vi "S4GUI_002.vi"(7 "Tab ObsEng":enum32{"Obs", "CCD modes", "Eng"}(tab)) -> ()   [LabVIEW 2018] (continued)
                n2860 = call-dynamic "Read ref StatesQueue.vi"("error in (no error)"=w6117, "State Machine in"=w6116) -> ("error out"=w6127:errorcluster, "ref StatesQueue"=w6119:refnum<queue>, "State Machine out"=w6128:refnum<class "State Machine.lvclass">)  [unwired: 7 in]
                n2861 = Flush Queue(queue=w6119, error in (no error)=w6127) -> (queue out=w6118:refnum<queue>, error out=w6123:errorcluster)  [unwired: 1 out]
                n2862 = Enqueue Element(queue=w6118, element=u32 300 ("State"), error in (no error)=w6123) -> (queue out=w6126:refnum<queue>, error out=w6122:errorcluster)  [unwired: 1 in, 1 out]
                n2863 = Enqueue Element(queue=w6126, element=u32 60 ("State"), error in (no error)=w6122) -> (queue out=w6125:refnum<queue>, error out=w6124:errorcluster)  [unwired: 1 in, 1 out]
                n2864 = call-dynamic "Write ref StatesQueue.vi"("error in (no error)"=w6124, "ref StatesQueue"=w6125, "State Machine in"=w6128) -> ("error out"=w6114:errorcluster, "State Machine out"=w6115:refnum<class "State Machine.lvclass">)  [unwired: 7 in]
                n2865 = call-dynamic "Write State.vi"("error in (no error)"=w6114, "State"=0, "State Machine in"=w6115) -> ("error out"=w6131:errorcluster, "State Machine out"=w6134:refnum<class "State Machine.lvclass">)  [unwired: 7 in]
                n2866 = call-dynamic "Write State Machine.vi"("error in (no error)"=w6131, "State Machine.lvclass"=w6134, "Device in"=w6133) -> ("error out"=w6136:errorcluster, "Device out"=w6135:refnum<class "Channel.lvclass">)  [unwired: 7 in]
              }
            }
            n2867 = case shown="True" w5842 {
              tunnel: [w6087 w6107] -> w5884
              tunnel: [w6088 w6106] -> w5883
              tunnel: w5864 -> [w6088 w6105]
              tunnel: w5863 -> [w6087 w6104]
              frame False {
              }
              frame True {
                # "command WRITE_SETUP"
                # "command SET SUFFIX"
                n2868 = call-dynamic "Read State Machine.vi"("error in (no error)"=w6104, "Device in"=w6105) -> ("error out"=w6091:errorcluster, "State Machine.lvclass"=w6092:refnum<class "State Machine.lvclass">, "Device out"=w6109:refnum<class "Channel.lvclass">)  [unwired: 7 in]
                n2869 = call-dynamic "Read ref StatesQueue.vi"("error in (no error)"=w6091, "State Machine in"=w6092) -> ("error out"=w6102:errorcluster, "ref StatesQueue"=w6094:refnum<queue>, "State Machine out"=w6103:refnum<class "State Machine.lvclass">)  [unwired: 7 in]
                n2870 = Flush Queue(queue=w6094, error in (no error)=w6102) -> (queue out=w6093:refnum<queue>, error out=w6098:errorcluster)  [unwired: 1 out]
                n2871 = Enqueue Element(queue=w6093, element=u32 300 ("State"), error in (no error)=w6098) -> (queue out=w6101:refnum<queue>, error out=w6097:errorcluster)  [unwired: 1 in, 1 out]
                n2872 = Enqueue Element(queue=w6101, element=u32 60 ("State"), error in (no error)=w6097) -> (queue out=w6100:refnum<queue>, error out=w6099:errorcluster)  [unwired: 1 in, 1 out]
                n2873 = call-dynamic "Write ref StatesQueue.vi"("error in (no error)"=w6099, "ref StatesQueue"=w6100, "State Machine in"=w6103) -> ("error out"=w6089:errorcluster, "State Machine out"=w6090:refnum<class "State Machine.lvclass">)  [unwired: 7 in]
                n2874 = call-dynamic "Write State.vi"("error in (no error)"=w6089, "State"=0, "State Machine in"=w6090) -> ("error out"=w6111:errorcluster, "State Machine out"=w6108:refnum<class "State Machine.lvclass">)  [unwired: 7 in]
                n2875 = call-dynamic "Write State Machine.vi"("error in (no error)"=w6111, "State Machine.lvclass"=w6108, "Device in"=w6109) -> ("error out"=w6107:errorcluster, "Device out"=w6106:refnum<class "Channel.lvclass">)  [unwired: 7 in]
              }
            }
            n2876 = call-dynamic "Write Channel.vi"("error in (no error)"=w6042, "Channel.lvclass"=w6043, "Acquisition in"=w6057) -> ("error out"=w6085:errorcluster, "Acquisition out"=w6086:refnum<class "Acquisition.lvclass">)  [unwired: 7 in]
            n2877 = call-dynamic "Write Channel.vi"("error in (no error)"=w6004, "Channel.lvclass"=w6003, "Acquisition in"=w5989) -> ("error out"=w6083:errorcluster, "Acquisition out"=w6084:refnum<class "Acquisition.lvclass">)  [unwired: 7 in]
            n2878 = call-dynamic "Write Channel.vi"("error in (no error)"=w5951, "Channel.lvclass"=w5950, "Acquisition in"=w5936) -> ("error out"=w6081:errorcluster, "Acquisition out"=w6082:refnum<class "Acquisition.lvclass">)  [unwired: 7 in]
            n2879 = call-dynamic "Write Channel.vi"("error in (no error)"=w5884, "Channel.lvclass"=w5883, "Acquisition in"=w5898) -> ("error out"=w6079:errorcluster, "Acquisition out"=w6080:refnum<class "Acquisition.lvclass">)  [unwired: 7 in]
          }
          frame "OBJECT", Default {
            # "nome do arquivo .cfg"
            # "seção no arquivo .cfg"
            # "open"
            # "nome do arquivo .cfg"
            # "seção no arquivo .cfg"
            # "open"
            # "nome do arquivo .cfg"
            # "seção no arquivo .cfg"
            # "open"
            # "nome do arquivo .cfg"
            # "seção no arquivo .cfg"
            # "open"
            # "OBJECT, DFLAT,SFLAT and FOCUS: Shutter automatically open and restore FRAME_TRANSFER."
            n2880 = call "Read connection.vi"("error in (no error)"=w6462, "Server in"=w6463) -> ("error out"=w6460:errorcluster, "connection"=w6227:bool, "Server out"=w6461:refnum<class "Acquisition.lvclass">)  [unwired: 7 in]
            n2881 = call "Read connection.vi"("error in (no error)"=w6448, "Server in"=w6449) -> ("error out"=w6454:errorcluster, "connection"=w6230:bool, "Server out"=w6455:refnum<class "Acquisition.lvclass">)  [unwired: 7 in]
            n2882 = call "Read connection.vi"("error in (no error)"=w6450, "Server in"=w6451) -> ("error out"=w6456:errorcluster, "connection"=w6229:bool, "Server out"=w6457:refnum<class "Acquisition.lvclass">)  [unwired: 7 in]
            n2883 = call "Read connection.vi"("error in (no error)"=w6452, "Server in"=w6453) -> ("error out"=w6458:errorcluster, "connection"=w6228:bool, "Server out"=w6459:refnum<class "Acquisition.lvclass">)  [unwired: 7 in]
            n2884 = call-dynamic "Read Channel.vi"("error in (no error)"=w6454, "Acquisition in"=w6455) -> ("error out"=w6281:errorcluster, "Channel.lvclass"=w6282:refnum<class "Channel.lvclass">, "Acquisition out"=w6283:refnum<class "Acquisition.lvclass">)  [unwired: 7 in]
            n2885 = call-dynamic "Read Channel.vi"("error in (no error)"=w6460, "Acquisition in"=w6461) -> ("error out"=w6440:errorcluster, "Channel.lvclass"=w6441:refnum<class "Channel.lvclass">, "Acquisition out"=w6442:refnum<class "Acquisition.lvclass">)  [unwired: 7 in]
            n2886 = call-dynamic "Read Channel.vi"("error in (no error)"=w6456, "Acquisition in"=w6457) -> ("error out"=w6325:errorcluster, "Channel.lvclass"=w6324:refnum<class "Channel.lvclass">, "Acquisition out"=w6323:refnum<class "Acquisition.lvclass">)  [unwired: 7 in]
            n2887 = call-dynamic "Read Channel.vi"("error in (no error)"=w6458, "Acquisition in"=w6459) -> ("error out"=w6378:errorcluster, "Channel.lvclass"=w6377:refnum<class "Channel.lvclass">, "Acquisition out"=w6376:refnum<class "Acquisition.lvclass">)  [unwired: 7 in]
            n2888 = call-dynamic "Read Interface.vi"("error in (no error)"=w6281, "Channel in"=w6282) -> ("error out"=w6249:errorcluster, "Interface.lvclass"=w6250:refnum<class "Interface.lvclass">, "Channel out"=w6246:refnum<class "Channel.lvclass">)  [unwired: 7 in]
            n2889 = call-dynamic "Read Interface.vi"("error in (no error)"=w6440, "Channel in"=w6441) -> ("error out"=w6402:errorcluster, "Interface.lvclass"=w6403:refnum<class "Interface.lvclass">, "Channel out"=w6392:refnum<class "Channel.lvclass">)  [unwired: 7 in]
            n2890 = call-dynamic "Read Interface.vi"("error in (no error)"=w6325, "Channel in"=w6324) -> ("error out"=w6299:errorcluster, "Interface.lvclass"=w6301:refnum<class "Interface.lvclass">, "Channel out"=w6296:refnum<class "Channel.lvclass">)  [unwired: 7 in]
            n2891 = call-dynamic "Read Interface.vi"("error in (no error)"=w6378, "Channel in"=w6377) -> ("error out"=w6352:errorcluster, "Interface.lvclass"=w6354:refnum<class "Interface.lvclass">, "Channel out"=w6349:refnum<class "Channel.lvclass">)  [unwired: 7 in]
            n2892 = call-dynamic "Read restoreExpTime.vi"("error in (no error)"=w6249, "Interface in"=w6250) -> ("error out"=w6248:errorcluster, "restoreExpTime"=w6251:bool, "Interface out"=w6247:refnum<class "Interface.lvclass">)  [unwired: 7 in]
            n2893 = call-dynamic "Read restoreExpTime.vi"("error in (no error)"=w6299, "Interface in"=w6301) -> ("error out"=w6298:errorcluster, "restoreExpTime"=w6297:bool, "Interface out"=w6300:refnum<class "Interface.lvclass">)  [unwired: 7 in]
            n2894 = call-dynamic "Read restoreExpTime.vi"("error in (no error)"=w6402, "Interface in"=w6403) -> ("error out"=w6400:errorcluster, "restoreExpTime"=w6399:bool, "Interface out"=w6401:refnum<class "Interface.lvclass">)  [unwired: 7 in]
            n2895 = call-dynamic "Read restoreExpTime.vi"("error in (no error)"=w6352, "Interface in"=w6354) -> ("error out"=w6351:errorcluster, "restoreExpTime"=w6350:bool, "Interface out"=w6353:refnum<class "Interface.lvclass">)  [unwired: 7 in]
            n2896 = case shown="True" w6251 {
              tunnel: w6247 -> [w6573 w6578]
              tunnel: [w6573 w6581] -> w6253
              tunnel: w6248 -> [w6572 w6577]
              tunnel: [w6572 w6580] -> w6252
              frame False {
              }
              frame True {
                n2897 = call-dynamic "Write restoreExpTime.vi"("error in (no error)"=w6577, "restoreExpTime"=FALSE, "Interface in"=w6578) -> ("error out"=w6575:errorcluster, "Interface out"=w6576:refnum<class "Interface.lvclass">)  [unwired: 7 in]
                n2898 = call-dynamic "Read prev ExpTime.vi"("error in (no error)"=w6575, "Interface in"=w6576) -> ("error out"=w6580:errorcluster, "prev ExpTime"=w6579:dbl, "Interface out"=w6581:refnum<class "Interface.lvclass">)  [unwired: 7 in]
                n2899 = property on="Exptime ch4" class="DigNum (strict)"("Value"=w6579) -> ()  [unwired: 2 in, 2 out]
              }
            }
            n2900 = case shown="True" w6297 {
              tunnel: w6300 -> [w6583 w6588]
              tunnel: [w6583 w6591] -> w6303
              tunnel: w6298 -> [w6582 w6587]
              tunnel: [w6582 w6590] -> w6302
              frame False {
              }
              frame True {
                n2901 = call-dynamic "Write restoreExpTime.vi"("error in (no error)"=w6587, "restoreExpTime"=FALSE, "Interface in"=w6588) -> ("error out"=w6585:errorcluster, "Interface out"=w6586:refnum<class "Interface.lvclass">)  [unwired: 7 in]
                n2902 = call-dynamic "Read prev ExpTime.vi"("error in (no error)"=w6585, "Interface in"=w6586) -> ("error out"=w6590:errorcluster, "prev ExpTime"=w6589:dbl, "Interface out"=w6591:refnum<class "Interface.lvclass">)  [unwired: 7 in]
                n2903 = property on="Exptime ch3" class="DigNum (strict)"("Value"=w6589) -> ()  [unwired: 2 in, 2 out]
              }
            }
            n2904 = case shown="True" w6399 {
              tunnel: w6401 -> [w6603 w6608]
              tunnel: [w6603 w6611] -> w6405
              tunnel: w6400 -> [w6602 w6606]
              tunnel: [w6602 w6610] -> w6404
              frame False {
              }
              frame True {
                n2905 = call-dynamic "Write restoreExpTime.vi"("error in (no error)"=w6606, "restoreExpTime"=FALSE, "Interface in"=w6608) -> ("error out"=w6605:errorcluster, "Interface out"=w6607:refnum<class "Interface.lvclass">)  [unwired: 7 in]
                n2906 = call-dynamic "Read prev ExpTime.vi"("error in (no error)"=w6605, "Interface in"=w6607) -> ("error out"=w6610:errorcluster, "prev ExpTime"=w6609:dbl, "Interface out"=w6611:refnum<class "Interface.lvclass">)  [unwired: 7 in]
                n2907 = property on="Exptime ch1" class="DigNum (strict)"("Value"=w6609) -> ()  [unwired: 2 in, 2 out]
              }
            }
            n2908 = case shown="True" w6350 {
              tunnel: w6353 -> [w6593 w6598]
              tunnel: [w6593 w6601] -> w6356
              tunnel: w6351 -> [w6592 w6597]
              tunnel: [w6592 w6600] -> w6355
              frame False {
              }
              frame True {
                n2909 = call-dynamic "Write restoreExpTime.vi"("error in (no error)"=w6597, "restoreExpTime"=FALSE, "Interface in"=w6598) -> ("error out"=w6595:errorcluster, "Interface out"=w6596:refnum<class "Interface.lvclass">)  [unwired: 7 in]
                n2910 = call-dynamic "Read prev ExpTime.vi"("error in (no error)"=w6595, "Interface in"=w6596) -> ("error out"=w6600:errorcluster, "prev ExpTime"=w6599:dbl, "Interface out"=w6601:refnum<class "Interface.lvclass">)  [unwired: 7 in]
                n2911 = property on="Exptime ch2" class="DigNum (strict)"("Value"=w6599) -> ()  [unwired: 2 in, 2 out]
              }
            }
            n2912 = call-dynamic "Read PREV_FT.vi"("error in (no error)"=w6252, "Interface in"=w6253) -> ("error out"=w6245:errorcluster, "PREV_FT"=w6254:bool, "Interface out"=w6243:refnum<class "Interface.lvclass">)  [unwired: 7 in]
            n2913 = call-dynamic "Read PREV_FT.vi"("error in (no error)"=w6355, "Interface in"=w6356) -> ("error out"=w6347:errorcluster, "PREV_FT"=w6357:bool, "Interface out"=w6346:refnum<class "Interface.lvclass">)  [unwired: 7 in]
            n2914 = call-dynamic "Read PREV_FT.vi"("error in (no error)"=w6302, "Interface in"=w6303) -> ("error out"=w6294:errorcluster, "PREV_FT"=w6304:bool, "Interface out"=w6293:refnum<class "Interface.lvclass">)  [unwired: 7 in]
            n2915 = call-dynamic "Read PREV_FT.vi"("error in (no error)"=w6404, "Interface in"=w6405) -> ("error out"=w6398:errorcluster, "PREV_FT"=w6406:bool, "Interface out"=w6397:refnum<class "Interface.lvclass">)  [unwired: 7 in]
            n2916 = call-dynamic "Read target cluster.vi"("error in (no error)"=w6245, "Channel in"=w6246) -> ("error out"=w6240:errorcluster, "target cluster"=w6244:T31, "Channel out"=w6242:refnum<class "Channel.lvclass">)  [unwired: 7 in]
            n2917 = Bundle By Name(cluster=w6244, "SHUTTER_MODE"=u8 1, "FRAME_TRANSFER"=w6254) -> (w6241:T31)
            n2918 = call-dynamic "Read target cluster.vi"("error in (no error)"=w6398, "Channel in"=w6392) -> ("error out"=w6393:errorcluster, "target cluster"=w6396:T31, "Channel out"=w6391:refnum<class "Channel.lvclass">)  [unwired: 7 in]
            n2919 = Bundle By Name(cluster=w6396, "SHUTTER_MODE"=u8 1, "FRAME_TRANSFER"=w6406) -> (w6395:T31)
            n2920 = call-dynamic "Read target cluster.vi"("error in (no error)"=w6347, "Channel in"=w6349) -> ("error out"=w6344:errorcluster, "target cluster"=w6348:T31, "Channel out"=w6342:refnum<class "Channel.lvclass">)  [unwired: 7 in]
            n2921 = Bundle By Name(cluster=w6348, "SHUTTER_MODE"=u8 1, "FRAME_TRANSFER"=w6357) -> (w6345:T31)
            n2922 = call-dynamic "Read target cluster.vi"("error in (no error)"=w6294, "Channel in"=w6296) -> ("error out"=w6291:errorcluster, "target cluster"=w6295:T31, "Channel out"=w6289:refnum<class "Channel.lvclass">)  [unwired: 7 in]
            n2923 = Bundle By Name(cluster=w6295, "SHUTTER_MODE"=u8 1, "FRAME_TRANSFER"=w6304) -> (w6292:T31)
            n2924 = call-dynamic "Write target cluster.vi"("error in (no error)"=w6240, "target cluster"=w6241, "Channel in"=w6242) -> ("error out"=w6239:errorcluster, "Channel out"=w6238:refnum<class "Channel.lvclass">)  [unwired: 7 in]
            n2925 = call-dynamic "Write target cluster.vi"("error in (no error)"=w6393, "target cluster"=w6395, "Channel in"=w6391) -> ("error out"=w6394:errorcluster, "Channel out"=w6390:refnum<class "Channel.lvclass">)  [unwired: 7 in]
            n2926 = call-dynamic "Write target cluster.vi"("error in (no error)"=w6344, "target cluster"=w6345, "Channel in"=w6342) -> ("error out"=w6343:errorcluster, "Channel out"=w6341:refnum<class "Channel.lvclass">)  [unwired: 7 in]
            n2927 = call-dynamic "Write target cluster.vi"("error in (no error)"=w6291, "target cluster"=w6292, "Channel in"=w6289) -> ("error out"=w6290:errorcluster, "Channel out"=w6288:refnum<class "Channel.lvclass">)  [unwired: 7 in]
            n2928 = Flatten To String(anything=w6241, error in (no error)=w6239) -> (data string=w6280:string, error out=w6279:errorcluster)  [unwired: 2 in, 1 out]
            n2929 = Flatten To String(anything=w6395, error in (no error)=w6394) -> (data string=w6439:string, error out=w6438:errorcluster)  [unwired: 2 in, 1 out]
            n2930 = Flatten To String(anything=w6345, error in (no error)=w6343) -> (data string=w6379:string, error out=w6380:errorcluster)  [unwired: 2 in, 1 out]
            n2931 = Flatten To String(anything=w6292, error in (no error)=w6290) -> (data string=w6326:string, error out=w6327:errorcluster)  [unwired: 2 in, 1 out]
            n2932 = call "Write flatted cluster.vi"("error in (no error)"=w6279, "flatted cluster"=w6280, "Interface in"=w6243) -> ("error out"=w6276:errorcluster, "Interface out"=w6277:refnum<class "Interface.lvclass">)  [unwired: 7 in]
            n2933 = call "Write flatted cluster.vi"("error in (no error)"=w6438, "flatted cluster"=w6439, "Interface in"=w6397) -> ("error out"=w6435:errorcluster, "Interface out"=w6436:refnum<class "Interface.lvclass">)  [unwired: 7 in]
            n2934 = call "Write flatted cluster.vi"("error in (no error)"=w6380, "flatted cluster"=w6379, "Interface in"=w6346) -> ("error out"=w6383:errorcluster, "Interface out"=w6382:refnum<class "Interface.lvclass">)  [unwired: 7 in]
            n2935 = call "Write flatted cluster.vi"("error in (no error)"=w6327, "flatted cluster"=w6326, "Interface in"=w6293) -> ("error out"=w6330:errorcluster, "Interface out"=w6329:refnum<class "Interface.lvclass">)  [unwired: 7 in]
            n2936 = call-dynamic "Write Interface.vi"("error in (no error)"=w6435, "Interface.lvclass"=w6436, "Channel in"=w6390) -> ("error out"=w6433:errorcluster, "Channel out"=w6432:refnum<class "Channel.lvclass">)  [unwired: 7 in]
            n2937 = call-dynamic "Write Interface.vi"("error in (no error)"=w6276, "Interface.lvclass"=w6277, "Channel in"=w6238) -> ("error out"=w6274:errorcluster, "Channel out"=w6273:refnum<class "Channel.lvclass">)  [unwired: 7 in]
            n2938 = call-dynamic "Write Interface.vi"("error in (no error)"=w6383, "Interface.lvclass"=w6382, "Channel in"=w6341) -> ("error out"=w6385:errorcluster, "Channel out"=w6386:refnum<class "Channel.lvclass">)  [unwired: 7 in]
            n2939 = call-dynamic "Write Interface.vi"("error in (no error)"=w6330, "Interface.lvclass"=w6329, "Channel in"=w6288) -> ("error out"=w6332:errorcluster, "Channel out"=w6333:refnum<class "Channel.lvclass">)  [unwired: 7 in]
            n2940 = call "Write section_name.vi"("error in (no error)"=w6433, "section_name"="CCD_ACS1", "Channel in"=w6432) -> ("error out"=w6434:errorcluster, "Channel out"=w6429:refnum<class "Channel.lvclass">)  [unwired: 7 in]
            n2941 = call "Write section_name.vi"("error in (no error)"=w6274, "section_name"="CCD_ACS4", "Channel in"=w6273) -> ("error out"=w6275:errorcluster, "Channel out"=w6270:refnum<class "Channel.lvclass">)  [unwired: 7 in]
            n2942 = call "Write section_name.vi"("error in (no error)"=w6385, "section_name"="CCD_ACS2", "Channel in"=w6386) -> ("error out"=w6384:errorcluster, "Channel out"=w6389:refnum<class "Channel.lvclass">)  [unwired: 7 in]
            n2943 = call "Write section_name.vi"("error in (no error)"=w6332, "section_name"="CCD_ACS3", "Channel in"=w6333) -> ("error out"=w6331:errorcluster, "Channel out"=w6336:refnum<class "Channel.lvclass">)  [unwired: 7 in]
            n2944 = call-dynamic "save config.vi"("error in (no error)"=w6434, "file config"="lastsaved.cfg", "Channel in"=w6429) -> ("error out"=w6410:errorcluster, "Channel out"=w6409:refnum<class "Channel.lvclass">)  [unwired: 7 in]
            n2945 = call-dynamic "save config.vi"("error in (no error)"=w6275, "file config"="lastsaved.cfg", "Channel in"=w6270) -> ("error out"=w6256:errorcluster, "Channel out"=w6258:refnum<class "Channel.lvclass">)  [unwired: 7 in]
            n2946 = call-dynamic "save config.vi"("error in (no error)"=w6384, "file config"="lastsaved.cfg", "Channel in"=w6389) -> ("error out"=w6359:errorcluster, "Channel out"=w6362:refnum<class "Channel.lvclass">)  [unwired: 7 in]
            n2947 = local read "Filter2"() -> (w6358:u8)
            n2948 = local read "Filter4"() -> (w6255:u8)
            n2949 = call-dynamic "save config.vi"("error in (no error)"=w6331, "file config"="lastsaved.cfg", "Channel in"=w6336) -> ("error out"=w6306:errorcluster, "Channel out"=w6307:refnum<class "Channel.lvclass">)  [unwired: 7 in]
            n2950 = local read "Filter1"() -> (w6411:u8)
            n2951 = local read "Filter3"() -> (w6305:u8)
            n2952 = call-dynamic "Write Filter.vi"("error in (no error)"=w6359, "Filter"=w6358, "Channel in"=w6362) -> ("error out"=w6375:errorcluster, "Channel out"=w6361:refnum<class "Channel.lvclass">)  [unwired: 7 in]
            n2953 = call-dynamic "Write Filter.vi"("error in (no error)"=w6256, "Filter"=w6255, "Channel in"=w6258) -> ("error out"=w6269:errorcluster, "Channel out"=w6257:refnum<class "Channel.lvclass">)  [unwired: 7 in]
            n2954 = call-dynamic "Write Filter.vi"("error in (no error)"=w6410, "Filter"=w6411, "Channel in"=w6409) -> ("error out"=w6426:errorcluster, "Channel out"=w6425:refnum<class "Channel.lvclass">)  [unwired: 7 in]
            n2955 = call-dynamic "Write Filter.vi"("error in (no error)"=w6306, "Filter"=w6305, "Channel in"=w6307) -> ("error out"=w6308:errorcluster, "Channel out"=w6321:refnum<class "Channel.lvclass">)  [unwired: 7 in]
            n2956 = call-dynamic "Read Interface.vi"("error in (no error)"=w6375, "Channel in"=w6361) -> ("error out"=w6372:errorcluster, "Interface.lvclass"=w6371:refnum<class "Interface.lvclass">, "Channel out"=w6360:refnum<class "Channel.lvclass">)  [unwired: 7 in]
            n2957 = call-dynamic "Read Interface.vi"("error in (no error)"=w6426, "Channel in"=w6425) -> ("error out"=w6422:errorcluster, "Interface.lvclass"=w6421:refnum<class "Interface.lvclass">, "Channel out"=w6415:refnum<class "Channel.lvclass">)  [unwired: 7 in]
            n2958 = call-dynamic "Read Interface.vi"("error in (no error)"=w6269, "Channel in"=w6257) -> ("error out"=w6268:errorcluster, "Interface.lvclass"=w6267:refnum<class "Interface.lvclass">, "Channel out"=w6233:refnum<class "Channel.lvclass">)  [unwired: 7 in]
            n2959 = call-dynamic "Read Interface.vi"("error in (no error)"=w6308, "Channel in"=w6321) -> ("error out"=w6311:errorcluster, "Interface.lvclass"=w6312:refnum<class "Interface.lvclass">, "Channel out"=w6322:refnum<class "Channel.lvclass">)  [unwired: 7 in]
            n2960 = call-dynamic "Write Suffix.vi"("error in (no error)"=w6372, "Suffix"=w6444, "Interface in"=w6371) -> ("error out"=w6363:errorcluster, "Interface out"=w6366:refnum<class "Interface.lvclass">)  [unwired: 7 in]
            n2961 = call-dynamic "Write Suffix.vi"("error in (no error)"=w6422, "Suffix"=w6444, "Interface in"=w6421) -> ("error out"=w6412:errorcluster, "Interface out"=w6416:refnum<class "Interface.lvclass">)  [unwired: 7 in]
            n2962 = call-dynamic "Write Suffix.vi"("error in (no error)"=w6268, "Suffix"=w6444, "Interface in"=w6267) -> ("error out"=w6259:errorcluster, "Interface out"=w6262:refnum<class "Interface.lvclass">)  [unwired: 7 in]
            n2963 = call-dynamic "Write Suffix.vi"("error in (no error)"=w6311, "Suffix"=w6444, "Interface in"=w6312) -> ("error out"=w6320:errorcluster, "Interface out"=w6317:refnum<class "Interface.lvclass">)  [unwired: 7 in]
            n2964 = call-dynamic "Write ObsType.vi"("error in (no error)"=w6412, "ObsType"=w6443, "Interface in"=w6416) -> ("error out"=w6413:errorcluster, "Interface out"=w6417:refnum<class "Interface.lvclass">)  [unwired: 7 in]
            n2965 = call-dynamic "Write ObsType.vi"("error in (no error)"=w6363, "ObsType"=w6443, "Interface in"=w6366) -> ("error out"=w6364:errorcluster, "Interface out"=w6367:refnum<class "Interface.lvclass">)  [unwired: 7 in]
            n2966 = call-dynamic "Write ObsType.vi"("error in (no error)"=w6259, "ObsType"=w6443, "Interface in"=w6262) -> ("error out"=w6260:errorcluster, "Interface out"=w6263:refnum<class "Interface.lvclass">)  [unwired: 7 in]
            n2967 = call-dynamic "Write ObsType.vi"("error in (no error)"=w6320, "ObsType"=w6443, "Interface in"=w6317) -> ("error out"=w6319:errorcluster, "Interface out"=w6316:refnum<class "Interface.lvclass">)  [unwired: 7 in]
            n2968 = call-dynamic "Write Object.vi"("error in (no error)"=w6413, "Object"=w6447, "Interface in"=w6417) -> ("error out"=w6414:errorcluster, "Interface out"=w6418:refnum<class "Interface.lvclass">)  [unwired: 7 in]
            n2969 = call-dynamic "Write Object.vi"("error in (no error)"=w6364, "Object"=w6447, "Interface in"=w6367) -> ("error out"=w6365:errorcluster, "Interface out"=w6368:refnum<class "Interface.lvclass">)  [unwired: 7 in]
            n2970 = call-dynamic "Write Object.vi"("error in (no error)"=w6260, "Object"=w6447, "Interface in"=w6263) -> ("error out"=w6261:errorcluster, "Interface out"=w6264:refnum<class "Interface.lvclass">)  [unwired: 7 in]
            n2971 = call-dynamic "Write Object.vi"("error in (no error)"=w6319, "Object"=w6447, "Interface in"=w6316) -> ("error out"=w6318:errorcluster, "Interface out"=w6315:refnum<class "Interface.lvclass">)  [unwired: 7 in]
            n2972 = call-dynamic "Write Comments.vi"("error in (no error)"=w6365, "Comments"=w6446, "Interface in"=w6368) -> ("error out"=w6369:errorcluster, "Interface out"=w6370:refnum<class "Interface.lvclass">)  [unwired: 7 in]
            n2973 = call-dynamic "Write Comments.vi"("error in (no error)"=w6414, "Comments"=w6446, "Interface in"=w6418) -> ("error out"=w6419:errorcluster, "Interface out"=w6420:refnum<class "Interface.lvclass">)  [unwired: 7 in]
            n2974 = call-dynamic "Write Comments.vi"("error in (no error)"=w6261, "Comments"=w6446, "Interface in"=w6264) -> ("error out"=w6265:errorcluster, "Interface out"=w6266:refnum<class "Interface.lvclass">)  [unwired: 7 in]
            n2975 = call-dynamic "Write Comments.vi"("error in (no error)"=w6318, "Comments"=w6446, "Interface in"=w6315) -> ("error out"=w6314:errorcluster, "Interface out"=w6313:refnum<class "Interface.lvclass">)  [unwired: 7 in]
            n2976 = call-dynamic "Write Observer.vi"("error in (no error)"=w6369, "Observer"=w6445, "Interface in"=w6370) -> ("error out"=w6374:errorcluster, "Interface out"=w6373:refnum<class "Interface.lvclass">)  [unwired: 7 in]
            n2977 = call-dynamic "Write Observer.vi"("error in (no error)"=w6419, "Observer"=w6445, "Interface in"=w6420) -> ("error out"=w6424:errorcluster, "Interface out"=w6423:refnum<class "Interface.lvclass">)  [unwired: 7 in]
            n2978 = call-dynamic "Write Observer.vi"("error in (no error)"=w6265, "Observer"=w6445, "Interface in"=w6266) -> ("error out"=w6231:errorcluster, "Interface out"=w6232:refnum<class "Interface.lvclass">)  [unwired: 7 in]
            n2979 = call-dynamic "Write Observer.vi"("error in (no error)"=w6314, "Observer"=w6445, "Interface in"=w6313) -> ("error out"=w6309:errorcluster, "Interface out"=w6310:refnum<class "Interface.lvclass">)  [unwired: 7 in]
            n2980 = call-dynamic "Write Interface.vi"("error in (no error)"=w6424, "Interface.lvclass"=w6423, "Channel in"=w6415) -> ("error out"=w6407:errorcluster, "Channel out"=w6408:refnum<class "Channel.lvclass">)  [unwired: 7 in]
            n2981 = call-dynamic "Write Interface.vi"("error in (no error)"=w6309, "Interface.lvclass"=w6310, "Channel in"=w6322) -> ("error out"=w6286:errorcluster, "Channel out"=w6287:refnum<class "Channel.lvclass">)  [unwired: 7 in]
            n2982 = call-dynamic "Write Interface.vi"("error in (no error)"=w6374, "Interface.lvclass"=w6373, "Channel in"=w6360) -> ("error out"=w6338:errorcluster, "Channel out"=w6340:refnum<class "Channel.lvclass">)  [unwired: 7 in]
            n2983 = call-dynamic "Write Interface.vi"("error in (no error)"=w6231, "Interface.lvclass"=w6232, "Channel in"=w6233) -> ("error out"=w6236:errorcluster, "Channel out"=w6237:refnum<class "Channel.lvclass">)  [unwired: 7 in]
            n2984 = case shown="True" w6227 {
              tunnel: [w6548 w6568] -> w6428
              tunnel: [w6547 w6567] -> w6427
              tunnel: w6408 -> [w6548 w6566]
              tunnel: w6407 -> [w6547 w6565]
              frame False {
              }
              frame True {
                n2985 = call-dynamic "Read State Machine.vi"("error in (no error)"=w6565, "Device in"=w6566) -> ("error out"=w6562:errorcluster, "State Machine.lvclass"=w6563:refnum<class "State Machine.lvclass">, "Device out"=w6570:refnum<class "Channel.lvclass">)  [unwired: 7 in]
                n2986 = call-dynamic "Read ref StatesQueue.vi"("error in (no error)"=w6562, "State Machine in"=w6563) -> ("error out"=w6560:errorcluster, "ref StatesQueue"=w6561:refnum<queue>, "State Machine out"=w6556:refnum<class "State Machine.lvclass">)  [unwired: 7 in]
                n2987 = Flush Queue(queue=w6561, error in (no error)=w6560) -> (queue out=w6559:refnum<queue>, error out=w6554:errorcluster)  [unwired: 1 out]
                n2988 = Enqueue Element(queue=w6559, element=u32 300 ("State"), error in (no error)=w6554) -> (queue out=w6558:refnum<queue>, error out=w6553:errorcluster)  [unwired: 1 in, 1 out]
                n2989 = Enqueue Element(queue=w6558, element=u32 60 ("State"), error in (no error)=w6553) -> (queue out=w6557:refnum<queue>, error out=w6555:errorcluster)  [unwired: 1 in, 1 out]
                n2990 = call-dynamic "Write ref StatesQueue.vi"("error in (no error)"=w6555, "ref StatesQueue"=w6557, "State Machine in"=w6556) -> ("error out"=w6551:errorcluster, "State Machine out"=w6552:refnum<class "State Machine.lvclass">)  [unwired: 7 in]
                n2991 = call-dynamic "Write State.vi"("error in (no error)"=w6551, "State"=0, "State Machine in"=w6552) -> ("error out"=w6571:errorcluster, "State Machine out"=w6569:refnum<class "State Machine.lvclass">)  [unwired: 7 in]
                n2992 = call-dynamic "Write State Machine.vi"("error in (no error)"=w6571, "State Machine.lvclass"=w6569, "Device in"=w6570) -> ("error out"=w6567:errorcluster, "Device out"=w6568:refnum<class "Channel.lvclass">)  [unwired: 7 in]
              }
            }
            n2993 = case shown="True" w6228 {
              tunnel: w6340 -> [w6523 w6528]
              tunnel: [w6523 w6526] -> w6339
              tunnel: w6338 -> [w6522 w6525]
              tunnel: [w6522 w6524] -> w6337
              frame False {
              }
              frame True {
                n2994 = call-dynamic "Read State Machine.vi"("error in (no error)"=w6525, "Device in"=w6528) -> ("error out"=w6542:errorcluster, "State Machine.lvclass"=w6543:refnum<class "State Machine.lvclass">, "Device out"=w6527:refnum<class "Channel.lvclass">)  [unwired: 7 in]
                n2995 = call-dynamic "Read ref StatesQueue.vi"("error in (no error)"=w6542, "State Machine in"=w6543) -> ("error out"=w6540:errorcluster, "ref StatesQueue"=w6541:refnum<queue>, "State Machine out"=w6536:refnum<class "State Machine.lvclass">)  [unwired: 7 in]
                n2996 = Flush Queue(queue=w6541, error in (no error)=w6540) -> (queue out=w6539:refnum<queue>, error out=w6534:errorcluster)  [unwired: 1 out]
                n2997 = Enqueue Element(queue=w6539, element=u32 300 ("State"), error in (no error)=w6534) -> (queue out=w6538:refnum<queue>, error out=w6533:errorcluster)  [unwired: 1 in, 1 out]
                n2998 = Enqueue Element(queue=w6538, element=u32 60 ("State"), error in (no error)=w6533) -> (queue out=w6537:refnum<queue>, error out=w6535:errorcluster)  [unwired: 1 in, 1 out]
                n2999 = call-dynamic "Write ref StatesQueue.vi"("error in (no error)"=w6535, "ref StatesQueue"=w6537, "State Machine in"=w6536) -> ("error out"=w6531:errorcluster, "State Machine out"=w6532:refnum<class "State Machine.lvclass">)  [unwired: 7 in]
                n3000 = call-dynamic "Write State.vi"("error in (no error)"=w6531, "State"=0, "State Machine in"=w6532) -> ("error out"=w6546:errorcluster, "State Machine out"=w6545:refnum<class "State Machine.lvclass">)  [unwired: 7 in]
                n3001 = call-dynamic "Write State Machine.vi"("error in (no error)"=w6546, "State Machine.lvclass"=w6545, "Device in"=w6527) -> ("error out"=w6524:errorcluster, "Device out"=w6526:refnum<class "Channel.lvclass">)  [unwired: 7 in]
              }
            }
            n3002 = case shown="True" w6229 {
              tunnel: w6287 -> [w6498 w6502]
              tunnel: w6286 -> [w6497 w6501]
              tunnel: [w6497 w6500] -> w6285
              tunnel: [w6498 w6499] -> w6284
              frame False {
              }
              frame True {
                n3003 = call-dynamic "Read State Machine.vi"("error in (no error)"=w6501, "Device in"=w6502) -> ("error out"=w6517:errorcluster, "State Machine.lvclass"=w6518:refnum<class "State Machine.lvclass">, "Device out"=w6503:refnum<class "Channel.lvclass">)  [unwired: 7 in]
                n3004 = call-dynamic "Read ref StatesQueue.vi"("error in (no error)"=w6517, "State Machine in"=w6518) -> ("error out"=w6515:errorcluster, "ref StatesQueue"=w6516:refnum<queue>, "State Machine out"=w6511:refnum<class "State Machine.lvclass">)  [unwired: 7 in]
                n3005 = Flush Queue(queue=w6516, error in (no error)=w6515) -> (queue out=w6514:refnum<queue>, error out=w6509:errorcluster)  [unwired: 1 out]
                n3006 = Enqueue Element(queue=w6514, element=u32 300 ("State"), error in (no error)=w6509) -> (queue out=w6513:refnum<queue>, error out=w6508:errorcluster)  [unwired: 1 in, 1 out]
                n3007 = Enqueue Element(queue=w6513, element=u32 60 ("State"), error in (no error)=w6508) -> (queue out=w6512:refnum<queue>, error out=w6510:errorcluster)  [unwired: 1 in, 1 out]
                n3008 = call-dynamic "Write ref StatesQueue.vi"("error in (no error)"=w6510, "ref StatesQueue"=w6512, "State Machine in"=w6511) -> ("error out"=w6506:errorcluster, "State Machine out"=w6507:refnum<class "State Machine.lvclass">)  [unwired: 7 in]
                n3009 = call-dynamic "Write State.vi"("error in (no error)"=w6506, "State"=0, "State Machine in"=w6507) -> ("error out"=w6521:errorcluster, "State Machine out"=w6520:refnum<class "State Machine.lvclass">)  [unwired: 7 in]
                n3010 = call-dynamic "Write State Machine.vi"("error in (no error)"=w6521, "State Machine.lvclass"=w6520, "Device in"=w6503) -> ("error out"=w6500:errorcluster, "Device out"=w6499:refnum<class "Channel.lvclass">)  [unwired: 7 in]
              }
            }
            n3011 = case shown="True" w6230 {
              tunnel: w6237 -> [w6473 w6481]
              tunnel: w6236 -> [w6472 w6480]
              tunnel: [w6472 w6479] -> w6235
              tunnel: [w6473 w6478] -> w6234
              frame False {
              }
              frame True {
                n3012 = call-dynamic "Read State Machine.vi"("error in (no error)"=w6480, "Device in"=w6481) -> ("error out"=w6494:errorcluster, "State Machine.lvclass"=w6477:refnum<class "State Machine.lvclass">, "Device out"=w6482:refnum<class "Channel.lvclass">)  [unwired: 7 in]
                n3013 = call-dynamic "Read ref StatesQueue.vi"("error in (no error)"=w6494, "State Machine in"=w6477) -> ("error out"=w6492:errorcluster, "ref StatesQueue"=w6493:refnum<queue>, "State Machine out"=w6476:refnum<class "State Machine.lvclass">)  [unwired: 7 in]
                n3014 = Flush Queue(queue=w6493, error in (no error)=w6492) -> (queue out=w6491:refnum<queue>, error out=w6487:errorcluster)  [unwired: 1 out]
                n3015 = Enqueue Element(queue=w6491, element=u32 300 ("State"), error in (no error)=w6487) -> (queue out=w6490:refnum<queue>, error out=w6486:errorcluster)  [unwired: 1 in, 1 out]
                n3016 = Enqueue Element(queue=w6490, element=u32 60 ("State"), error in (no error)=w6486) -> (queue out=w6489:refnum<queue>, error out=w6488:errorcluster)  [unwired: 1 in, 1 out]
                n3017 = call-dynamic "Write ref StatesQueue.vi"("error in (no error)"=w6488, "ref StatesQueue"=w6489, "State Machine in"=w6476) -> ("error out"=w6485:errorcluster, "State Machine out"=w6475:refnum<class "State Machine.lvclass">)  [unwired: 7 in]
                n3018 = call-dynamic "Write State.vi"("error in (no error)"=w6485, "State"=0, "State Machine in"=w6475) -> ("error out"=w6496:errorcluster, "State Machine out"=w6474:refnum<class "State Machine.lvclass">)  [unwired: 7 in]
                n3019 = call-dynamic "Write State Machine.vi"("error in (no error)"=w6496, "State Machine.lvclass"=w6474, "Device in"=w6482) -> ("error out"=w6479:errorcluster, "Device out"=w6478:refnum<class "Channel.lvclass">)  [unwired: 7 in]
              }
            }
            n3020 = call-dynamic "Write Channel.vi"("error in (no error)"=w6427, "Channel.lvclass"=w6428, "Acquisition in"=w6442) -> ("error out"=w6470:errorcluster, "Acquisition out"=w6471:refnum<class "Acquisition.lvclass">)  [unwired: 7 in]
            n3021 = call-dynamic "Write Channel.vi"("error in (no error)"=w6337, "Channel.lvclass"=w6339, "Acquisition in"=w6376) -> ("error out"=w6468:errorcluster, "Acquisition out"=w6469:refnum<class "Acquisition.lvclass">)  [unwired: 7 in]
            n3022 = call-dynamic "Write Channel.vi"("error in (no error)"=w6285, "Channel.lvclass"=w6284, "Acquisition in"=w6323) -> ("error out"=w6466:errorcluster, "Acquisition out"=w6467:refnum<class "Acquisition.lvclass">)  [unwired: 7 in]
            n3023 = call-dynamic "Write Channel.vi"("error in (no error)"=w6235, "Channel.lvclass"=w6234, "Acquisition in"=w6283) -> ("error out"=w6464:errorcluster, "Acquisition out"=w6465:refnum<class "Acquisition.lvclass">)  [unwired: 7 in]
          }
        }
        n3024 = call-dynamic "Write AcquisitionA.vi"("error in (no error)"=w5412, "Acquisition.lvclass"=w5413, "S4ACS_GUI in"=w5414) -> ("error out"=w5404:errorcluster, "S4ACS_GUI out"=w5408:refnum<class "S4GUI.lvclass">)  [unwired: 7 in]
        n3025 = call "Write AcquisitionB.vi"("error in (no error)"=w5409, "Acquisition.lvclass"=w5410, "S4ACS_GUI in"=w5408) -> ("error out"=w5403:errorcluster, "S4ACS_GUI out"=w5407:refnum<class "S4GUI.lvclass">)  [unwired: 7 in]
        n3026 = call-dynamic "Write AcquisitionC.vi"("error in (no error)"=w5398, "Acquisition.lvclass"=w5399, "S4ACS_GUI in"=w5407) -> ("error out"=w5402:errorcluster, "S4ACS_GUI out"=w5406:refnum<class "S4GUI.lvclass">)  [unwired: 7 in]
        n3027 = call-dynamic "Write AcquisitionD.vi"("error in (no error)"=w5396, "Acquisition.lvclass"=w5397, "S4ACS_GUI in"=w5406) -> ("error out"=w5401:errorcluster, "S4ACS_GUI out"=w5405:refnum<class "S4GUI.lvclass">)  [unwired: 7 in]
        n3028 = Merge Errors(w5404, w5403, w5402, w5401) -> (w5400:errorcluster)
        n3029 = call "Write cfg file.vi"("error in (no error)"=w5400, "cfg file"="lastsaved.cfg", "S4ACS_GUI in"=w5405) -> ("error out"=w5356:errorcluster, "S4ACS_GUI out"=w5357:refnum<class "S4GUI.lvclass">)  [unwired: 7 in]
        n3030 = disable-structure shown="Enabled" {
          disable-tunnel: w5357 -> [w5418 w5453]
          disable-tunnel: w5356 -> [w5417 w5452]
          disable-tunnel: [w5416 w5453] -> w5355
          disable-tunnel: [w5415 w5452] -> w5354
          frame Disabled {
            # "Este código passou para o evento \"Timeout\" (executa sempre)"
            # "1a vez FOTOM (F)"
            # "1a vez POLAR (F)"
            n3031 = call "Read Instrument.lvclass.vi"("error in (no error)"=w5417, "S4ACS_GUI in"=w5418) -> ("error out"=w5420:errorcluster, "Instrument.lvclass"=w5421:refnum<class "Instrument.lvclass">, "S4ACS_GUI out"=w5416:refnum<class "S4GUI.lvclass">)  [unwired: 7 in]
            n3032 = call-dynamic "Read mode.vi"("error in (no error)"=w5420, "Instrument in"=w5421) -> ("error out"=w5415:errorcluster, "mode"=w5419:bool)  [unwired: 7 in, 1 out]
            n3033 = while {
              tunnel: w5419 -> [w5426]
              shift-right: [w5422] -> _
              shift-left: _ -> [w5425]
              shift-right: [w5423] -> _
              shift-left: _ -> [w5424]
              stop <- TRUE stop-if-true
              # "Valores default para procedimento\nde ajuste de foco do telescópio"
              n3034 = case shown="True" w5426 {
                tunnel: w5425 -> [w5428 w5443]
                tunnel: [w5429 w5442] -> w5422
                tunnel: w5424 -> [w5431 w5441]
                tunnel: [w5430 w5440] -> w5423
                frame True {
                  # "polarimetria"
                  n3035 = case shown="False" w5431 {
                    selector: w5431 -> [w5435 w5439]
                    tunnel: [w5434 w5439] -> w5430
                    tunnel: [FALSE FALSE] -> w5429
                    tunnel: w5428 -> [_ _]
                    frame False {
                      w5432 = 12900
                      n3036 = local write "Start focus"(w5432) -> ()
                      n3037 = local write "Target focus"(w5432) -> ()
                      n3038 = local write "Step focus"(80) -> ()
                      n3039 = local write "#steps"(11) -> ()
                      n3040 = Not(x=w5435) -> (.not. x?=w5434:bool)
                    }
                    frame True {
                    }
                  }
                }
                frame False {
                  # "fotometria"
                  n3041 = case shown="False" w5443 {
                    selector: w5443 -> [w5446 w5451]
                    tunnel: [w5445 w5451] -> w5442
                    tunnel: w5441 -> [_ _]
                    tunnel: [FALSE FALSE] -> w5440
                    frame False {
                      w5444 = 13400
                      n3042 = local write "Start focus"(w5444) -> ()
                      n3043 = local write "Step focus"(100) -> ()
                      n3044 = local write "Target focus"(w5444) -> ()
                      n3045 = local write "#steps"(11) -> ()
                      n3046 = Not(x=w5446) -> (.not. x?=w5445:bool)
                    }
                    frame True {
                    }
                  }
                }
              }
            }
          }
          frame Enabled {
          }
        }
      }
      event "set keywords", "set Observer": Value Change {
        # "SET suffix e publica os outros campos da aba selecionada."
        n3047 = event-data() -> ()  [unwired: 1 in, 1 out]
        n3048 = local read "Tab Acq Type"() -> (w6750:T1)
        n3049 = case shown="\"OBJECT\", Default" w6750 {
          tunnel: ["OBJECT" "FLAT" "FLAT" "DARK" "ZERO" "FOCUS"] -> w6729
          tunnel: [w6831 w6835 w6839 w6843 w6847 w6852] -> w6730
          tunnel: [w6830 w6834 w6838 w6842 w6846 w6851] -> w6724
          tunnel: [w6829 w6833 w6837 w6841 w6845 w6850] -> w6723
          tunnel: [_ _ _ _ _ TRUE] -> _
          frame "OBJECT", Default {
            n3050 = local read "OBJECT Comments"() -> (w6829:string)
            n3051 = local read "Object_obj"() -> (w6831:string)
            n3052 = local read "object suffix"() -> (w6830:string)
          }
          frame "DFLAT" {
            n3053 = local read "DFLAT Comments"() -> (w6833:string)
            n3054 = local read "Object_dflat"() -> (w6835:string)
            n3055 = local read "dflat suffix"() -> (w6834:string)
          }
          frame "SFLAT" {
            n3056 = local read "SFLAT Comments"() -> (w6837:string)
            n3057 = local read "Object_sflat"() -> (w6839:string)
            n3058 = local read "sflat suffix"() -> (w6838:string)
          }
          frame "DARK" {
            n3059 = local read "DARK Comments"() -> (w6841:string)
            n3060 = local read "Object_dark"() -> (w6843:string)
            n3061 = local read "dark suffix"() -> (w6842:string)
          }
          frame "ZERO" {
            n3062 = local read "ZERO Comments"() -> (w6845:string)
            n3063 = local read "Object_zero"() -> (w6847:string)
            n3064 = local read "zero suffix"() -> (w6846:string)
          }
          frame "FOCUS" {
            n3065 = local read "FOCUS Comments"() -> (w6850:string)
            n3066 = local read "Object_focus"() -> (w6852:string)
            n3067 = local read "focus suffix"() -> (w6851:string)
          }
        }
        n3068 = call-dynamic "Write User Event.vi"("error in (no error)"=w6718, "User Event"="SET KEYWORDS CLICKED (Obsever, ProjectID, Object, Comments) ", "S4GUI in"=w6719) -> ("error out"=w6716:errorcluster, "S4GUI out"=w6717:refnum<class "S4GUI.lvclass">)  [unwired: 7 in]
        n3069 = call-dynamic "Read Publisher.lvclass.vi"("error in (no error)"=w6716, "S4GUI in"=w6717) -> ("error out"=w6740:errorcluster, "Publisher.lvclass"=w6736:refnum<class "Publisher.lvclass">, "S4GUI out"=w6741:refnum<class "S4GUI.lvclass">)  [unwired: 7 in]
        n3070 = call-dynamic "Write object.vi"("error in (no error)"=w6740, "object"=w6730, "Publisher in"=w6736) -> ("error out"=w6739:errorcluster, "Publisher out"=w6735:refnum<class "Publisher.lvclass">)  [unwired: 7 in]
        n3071 = call-dynamic "Write obstype.vi"("error in (no error)"=w6739, "obstype"=w6729, "Publisher in"=w6735) -> ("error out"=w6738:errorcluster, "Publisher out"=w6734:refnum<class "Publisher.lvclass">)  [unwired: 7 in]
        n3072 = call-dynamic "Write observer.vi"("error in (no error)"=w6738, "observer"=w6728, "Publisher in"=w6734) -> ("error out"=w6737:errorcluster, "Publisher out"=w6733:refnum<class "Publisher.lvclass">)  [unwired: 7 in]
        n3073 = call-dynamic "Write projid.vi"("error in (no error)"=w6737, "projid"=w6727, "Publisher in"=w6733) -> ("error out"=w6722:errorcluster, "Publisher out"=w6721:refnum<class "Publisher.lvclass">)  [unwired: 7 in]
        n3074 = call-dynamic "Write comments.vi"("error in (no error)"=w6722, "comments"=w6723, "Publisher in"=w6721) -> ("error out"=w6726:errorcluster, "Publisher out"=w6725:refnum<class "Publisher.lvclass">)  [unwired: 7 in]
        n3075 = call-dynamic "Write Publisher.lvclass.vi"("error in (no error)"=w6726, "Publisher.lvclass"=w6725, "S4GUI in"=w6741) -> ("error out"=w6731:errorcluster, "S4GUI out"=w6732:refnum<class "S4GUI.lvclass">)  [unwired: 7 in]
        n3076 = call-dynamic "Read AcquisitionC.vi"("error in (no error)"=w6731, "S4ACS_GUI in"=w6732) -> ("error out"=w6754:errorcluster, "Acquisition.lvclass"=w6755:refnum<class "Acquisition.lvclass">)  [unwired: 7 in, 1 out]
        n3077 = call-dynamic "Read AcquisitionA.vi"("error in (no error)"=w6731, "S4ACS_GUI in"=w6732) -> ("error out"=w6758:errorcluster, "Acquisition.lvclass"=w6759:refnum<class "Acquisition.lvclass">, "S4ACS_GUI out"=w6780:refnum<class "S4GUI.lvclass">)  [unwired: 7 in]
        n3078 = call "Read AcquisitionB.vi"("error in (no error)"=w6731, "S4ACS_GUI in"=w6732) -> ("error out"=w6756:errorcluster, "Acquisition.lvclass"=w6757:refnum<class "Acquisition.lvclass">)  [unwired: 7 in, 1 out]
        n3079 = call-dynamic "Read AcquisitionD.vi"("error in (no error)"=w6731, "S4ACS_GUI in"=w6732) -> ("error out"=w6752:errorcluster, "Acquisition.lvclass"=w6753:refnum<class "Acquisition.lvclass">)  [unwired: 7 in, 1 out]
        n3080 = call-dynamic "Read enabled.vi"("error in (no error)"=w6754, "Server in"=w6755) -> ("error out"=w6744:errorcluster, "enabled"=w6638:bool, "Server out"=w6745:refnum<class "Acquisition.lvclass">)  [unwired: 7 in]
        n3081 = call-dynamic "Read enabled.vi"("error in (no error)"=w6752, "Server in"=w6753) -> ("error out"=w6742:errorcluster, "enabled"=w6612:bool, "Server out"=w6743:refnum<class "Acquisition.lvclass">)  [unwired: 7 in]
        n3082 = call-dynamic "Read enabled.vi"("error in (no error)"=w6756, "Server in"=w6757) -> ("error out"=w6746:errorcluster, "enabled"=w6664:bool, "Server out"=w6747:refnum<class "Acquisition.lvclass">)  [unwired: 7 in]
        n3083 = call-dynamic "Read enabled.vi"("error in (no error)"=w6758, "Server in"=w6759) -> ("error out"=w6748:errorcluster, "enabled"=w6690:bool, "Server out"=w6749:refnum<class "Acquisition.lvclass">)  [unwired: 7 in]
        n3084 = call-dynamic "Read Channel.vi"("error in (no error)"=w6746, "Acquisition in"=w6747) -> ("error out"=w6669:errorcluster, "Channel.lvclass"=w6670:refnum<class "Channel.lvclass">, "Acquisition out"=w6687:refnum<class "Acquisition.lvclass">)  [unwired: 7 in]
        n3085 = call-dynamic "Read Channel.vi"("error in (no error)"=w6742, "Acquisition in"=w6743) -> ("error out"=w6617:errorcluster, "Channel.lvclass"=w6618:refnum<class "Channel.lvclass">, "Acquisition out"=w6637:refnum<class "Acquisition.lvclass">)  [unwired: 7 in]
        n3086 = call-dynamic "Read Channel.vi"("error in (no error)"=w6744, "Acquisition in"=w6745) -> ("error out"=w6643:errorcluster, "Channel.lvclass"=w6644:refnum<class "Channel.lvclass">, "Acquisition out"=w6661:refnum<class "Acquisition.lvclass">)  [unwired: 7 in]
        n3087 = call-dynamic "Read Channel.vi"("error in (no error)"=w6748, "Acquisition in"=w6749) -> ("error out"=w6695:errorcluster, "Channel.lvclass"=w6696:refnum<class "Channel.lvclass">, "Acquisition out"=w6715:refnum<class "Acquisition.lvclass">)  [unwired: 7 in]
        n3088 = To Lower Case(string=w6724) -> (all lower case string=w6751:string)
        n3089 = local read "Filter2"() -> (w6671:u8)
        n3090 = local read "Filter4"() -> (w6619:u8)
        n3091 = local read "Filter3"() -> (w6645:u8)
        n3092 = local read "Filter1"() -> (w6699:u8)
        n3093 = call-dynamic "Write Filter.vi"("error in (no error)"=w6617, "Filter"=w6619, "Channel in"=w6618) -> ("error out"=w6634:errorcluster, "Channel out"=w6623:refnum<class "Channel.lvclass">)  [unwired: 7 in]
        n3094 = call-dynamic "Write Filter.vi"("error in (no error)"=w6669, "Filter"=w6671, "Channel in"=w6670) -> ("error out"=w6686:errorcluster, "Channel out"=w6675:refnum<class "Channel.lvclass">)  [unwired: 7 in]
        n3095 = call-dynamic "Write Filter.vi"("error in (no error)"=w6643, "Filter"=w6645, "Channel in"=w6644) -> ("error out"=w6648:errorcluster, "Channel out"=w6659:refnum<class "Channel.lvclass">)  [unwired: 7 in]
        n3096 = call-dynamic "Write Filter.vi"("error in (no error)"=w6695, "Filter"=w6699, "Channel in"=w6696) -> ("error out"=w6712:errorcluster, "Channel out"=w6711:refnum<class "Channel.lvclass">)  [unwired: 7 in]
        n3097 = call-dynamic "Read Interface.vi"("error in (no error)"=w6634, "Channel in"=w6623) -> ("error out"=w6633:errorcluster, "Interface.lvclass"=w6632:refnum<class "Interface.lvclass">, "Channel out"=w6622:refnum<class "Channel.lvclass">)  [unwired: 7 in]
        n3098 = call-dynamic "Read Interface.vi"("error in (no error)"=w6686, "Channel in"=w6675) -> ("error out"=w6685:errorcluster, "Interface.lvclass"=w6684:refnum<class "Interface.lvclass">, "Channel out"=w6674:refnum<class "Channel.lvclass">)  [unwired: 7 in]
        n3099 = call-dynamic "Read Interface.vi"("error in (no error)"=w6648, "Channel in"=w6659) -> ("error out"=w6649:errorcluster, "Interface.lvclass"=w6650:refnum<class "Interface.lvclass">, "Channel out"=w6660:refnum<class "Channel.lvclass">)  [unwired: 7 in]
        n3100 = call-dynamic "Read Interface.vi"("error in (no error)"=w6712, "Channel in"=w6711) -> ("error out"=w6710:errorcluster, "Interface.lvclass"=w6709:refnum<class "Interface.lvclass">, "Channel out"=w6703:refnum<class "Channel.lvclass">)  [unwired: 7 in]
        n3101 = call-dynamic "Write Suffix.vi"("error in (no error)"=w6710, "Suffix"=w6751, "Interface in"=w6709) -> ("error out"=w6700:errorcluster, "Interface out"=w6704:refnum<class "Interface.lvclass">)  [unwired: 7 in]
        n3102 = call-dynamic "Write Suffix.vi"("error in (no error)"=w6633, "Suffix"=w6751, "Interface in"=w6632) -> ("error out"=w6624:errorcluster, "Interface out"=w6627:refnum<class "Interface.lvclass">)  [unwired: 7 in]
